vi "Set Home.vi"(8 "Error In":errorcluster, 11 "VISA resource in":refnum<visa-resource-name>) -> (0 "Error Out":errorcluster, 3 "VISA resource out":refnum<visa-resource-name>)   [LabVIEW 2014, in "Motor manager.lvlib"]
uses:
  Motor manager.lvlib
  Typedef/Commands.ctl
  Cmd to Byte Array (Sgl).vi
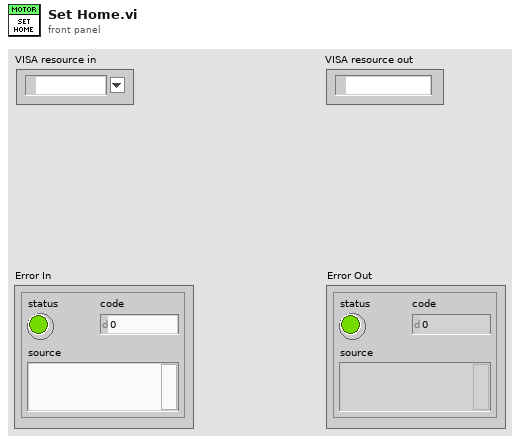
[diagram p1: front panel]
types:
  T1 = typedef "Motor manager.lvlib/Commands.ctl" = enum16{"None", "Set motor", "Set distance", "Set speed", "Set Move Type", "Set IM Idle Time", "Set N cycles", "Start", "Stop", "Stop and Release", "Set Home", "Find Home", "Move Forward", "Move Backward"}
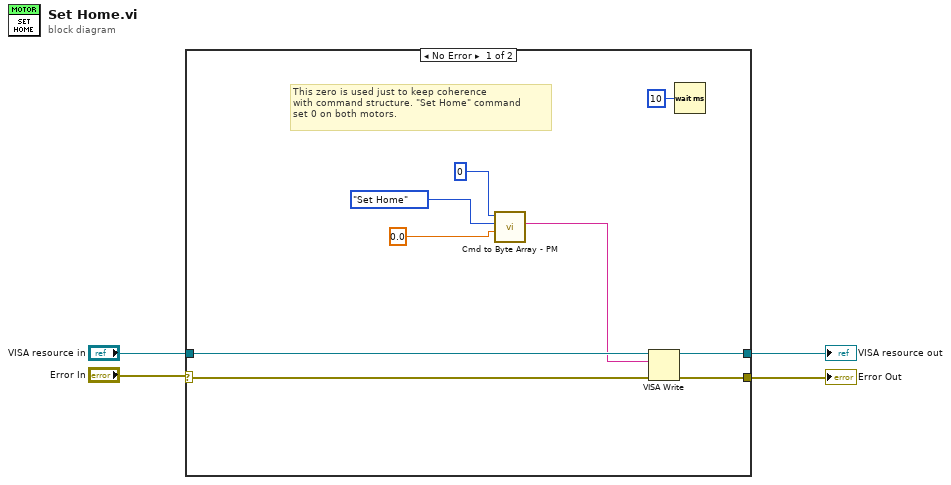
[diagram p0: block diagram]
diagram:
  n1 = case shown="No Error" "Error In" {
    selector: "Error In" -> [w10 w15]
    tunnel: "VISA resource in" -> [w11 w14]
    tunnel: [w13 w15] -> w2
    tunnel: [w12 w14] -> w1
    frame No Error {
      # "This zero is used just to keep coherence\nwith command structure. \"Set Home\" command\nset 0 on both motors."
      n2 = call-poly "Cmd to Byte Array - PM.vi"("Parameter"=sgl 0.0, "Commands"=Commands."Set Home", "Motor index"=u8 0) -> ("Byte string"=w8:string)  [unwired: 8 in]
      n3 = VISA Write(VISA resource name=w11, write buffer=w8, error in (no error)=w10) -> (VISA resource name out=w12:refnum<visa-resource-name>, error out=w13:errorcluster)  [unwired: 1 out]
      n4 = Wait (ms)(milliseconds to wait=u32 10) -> ()  [unwired: 1 out]
    }
    frame Error {
    }
  }
  "Error Out" <- w2
  "VISA resource out" <- w1
